vi "GetDirection.vi"(8 "error in (no error)":errorcluster, 11 "Snake in":refnum<class "SnakeGame.lvclass">) -> (0 "error out":errorcluster, 3 "Snake out":refnum<class "SnakeGame.lvclass">)   [LabVIEW 2019, in "RT_Game.lvlib" / "SnakeGame.lvclass"]
uses:
  SnakeGame.lvclass
  C:/Users/FreshBob/Dropbox/VIs/myRIO_GameConsole/RT/RT_Game/Game/Game.lvclass
  Game/Game.lvclass/Game.ctl
  SnakeGame.lvclass/SnakeGame.ctl
  Game/Game.lvclass
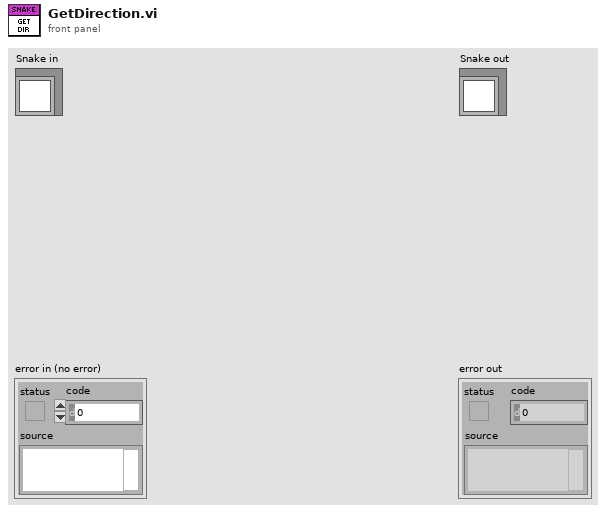
[diagram p1: front panel]
types:
  T1 = cluster{"Controls_1":cluster{"DirectionX":i8, "DirectionY":i8, "Button1":bool, "Button2":bool}, "Controls_2":cluster{"DirectionX":i8, "DirectionY":i8, "Button1":bool, "Button2":bool}, "SystemButton":bool}
  T2 = typedef "RT_Game.lvlib/SnakeGame.lvclass/Direction.ctl" = enum16{"Up", "Left", "Down", "Right"}
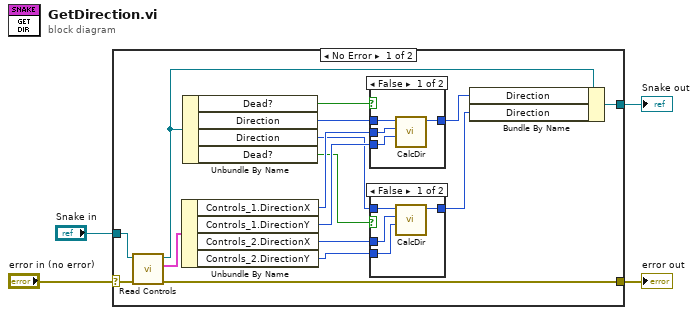
[diagram p0: block diagram]
diagram:
  n1 = case shown="No Error" "error in (no error)" {
    selector: "error in (no error)" -> [w20 w32]
    tunnel: [w19 w32] -> w3
    tunnel: [w14 w31] -> w1
    tunnel: "Snake in" -> [w18 w31]
    frame No Error {
      n2 = call "Read Controls.vi"("error in (no error)"=w20, "Game in"=w18) -> ("error out"=w19:errorcluster, "Controls"=w17:T1, "Game out"=w12:refnum<class "SnakeGame.lvclass">)  [unwired: 7 in]
      n3 = Unbundle By Name(w17) -> ("Controls_1.DirectionX"=w16:i8, "Controls_1.DirectionY"=w15:i8, "Controls_2.DirectionX"=w8:i8, "Controls_2.DirectionY"=w7:i8)
      n4 = Unbundle By Name(w12) -> ("Dead?"=w6:bool, "Direction"=w11:T2, "Direction"=w10:T2, "Dead?"=w5:bool)
      n5 = case shown="False" w6 {
        tunnel: w16 -> [w24 _]
        tunnel: w15 -> [w23 _]
        tunnel: [w22 w25] -> w13
        tunnel: w11 -> [w21 w25]
        frame False {
          n6 = call "CalcDir.vi"("DirectionY"=w23, "DirectionX"=w24, "Direction in"=w21) -> ("Direction out"=w22:T2)  [unwired: 8 in]
        }
        frame True {
        }
      }
      n7 = case shown="False" w5 {
        tunnel: w10 -> [w29 w30]
        tunnel: [w28 w30] -> w9
        tunnel: w8 -> [w27 _]
        tunnel: w7 -> [w26 _]
        frame False {
          n8 = call "CalcDir.vi"("DirectionY"=w26, "DirectionX"=w27, "Direction in"=w29) -> ("Direction out"=w28:T2)  [unwired: 8 in]
        }
        frame True {
        }
      }
      n9 = Bundle By Name(cluster=w12, "Direction"=w13, "Direction"=w9) -> (w14:refnum<class "SnakeGame.lvclass">)
    }
    frame Error {
    }
  }
  "error out" <- w3
  "Snake out" <- w1
